vi "FaceDLControl.vi"(0 "Data In":T7 caption="Données en entrée", 2 "Display State In":T5 caption="État d'affichage en entrée", 3 "Container State":T6 caption="État du conteneur") -> (6 "Data Out":T7 caption="Données en sortie", 7 "Display State Out":T5 caption="État d'affichage en sortie", 8 "Action":T4)   [LabVIEW 2015, in "ControlDL.xctl"]
uses:
  ControlDL.xctl
  <vilib>/_xctls/Action.ctl
  <vilib>/_xctls/XControlSupport.lvlib
  <vilib>/_xctls/Container State.ctl
  DataDLControl.ctl
  stateDLControl.ctl
  controls/DLSD.ctl
  controls/DLlongVerSD.ctl
panel:
  in  "param":T1={"Short"={"min"=-100.0, "max"=48.0, "real pos"=-48.0}, "Long"={"min"=-900.0, "max"=100.0, "real pos"=-100.0}}
  in  "Enable":bool
  in  "pos long":dbl caption="pos, mm"
  in  "DL_long":T2=1.0 min=0.0 max=1.0 scale=-0.1..1.2 scale format="%.2f"
  in  "pos short":dbl caption="pos,mm"
  in  "DL_short":T3=1.0 min=0.0 max=1.0 scale format="%#_6f"
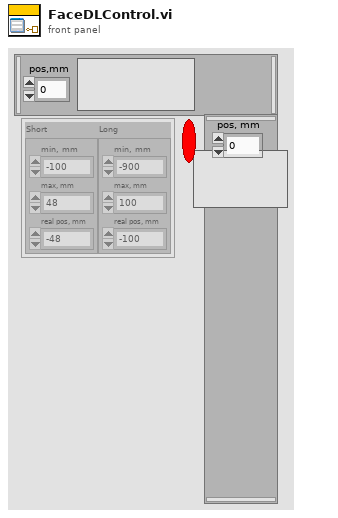
[diagram p1: front panel]
types:
  T1 = cluster{"Short":cluster{"min":dbl, "max":dbl, "real pos":dbl}, "Long":cluster{"min":dbl, "max":dbl, "real pos":dbl}}
  T2 = typedef "DLlongVerSD.ctl" = dbl
  T3 = typedef "DLSD.ctl" = dbl
  T4 = typedef "XControlSupport.lvlib/Action.ctl" = cluster{"Data Changed?":bool, "State Changed?":bool, "Action Name":string}
  T5 = typedef "ControlDL.xctl/stateDLControl.ctl" = cluster{"param":cluster{"Short":cluster{"min":dbl, "max":dbl, "real pos":dbl}, "Long":cluster{"min":dbl, "max":dbl, "real pos":dbl}}, "pos short":dbl, "pos Long":dbl, "DLmove_short":refnum<user-event>, "DLmove_long":refnum<user-event>}
  T6 = typedef "XControlSupport.lvlib/Container State.ctl" = cluster{"Indicator?":bool, "Run Mode?":bool, " Refnum":refnum<vi>}
  T7 = typedef "ControlDL.xctl/DataDLControl.ctl" = cluster{"pos short":dbl, "pos long":dbl}
  T8 = enum8{"Enabled", "Disabled", "Disabled and Grayed Out"}
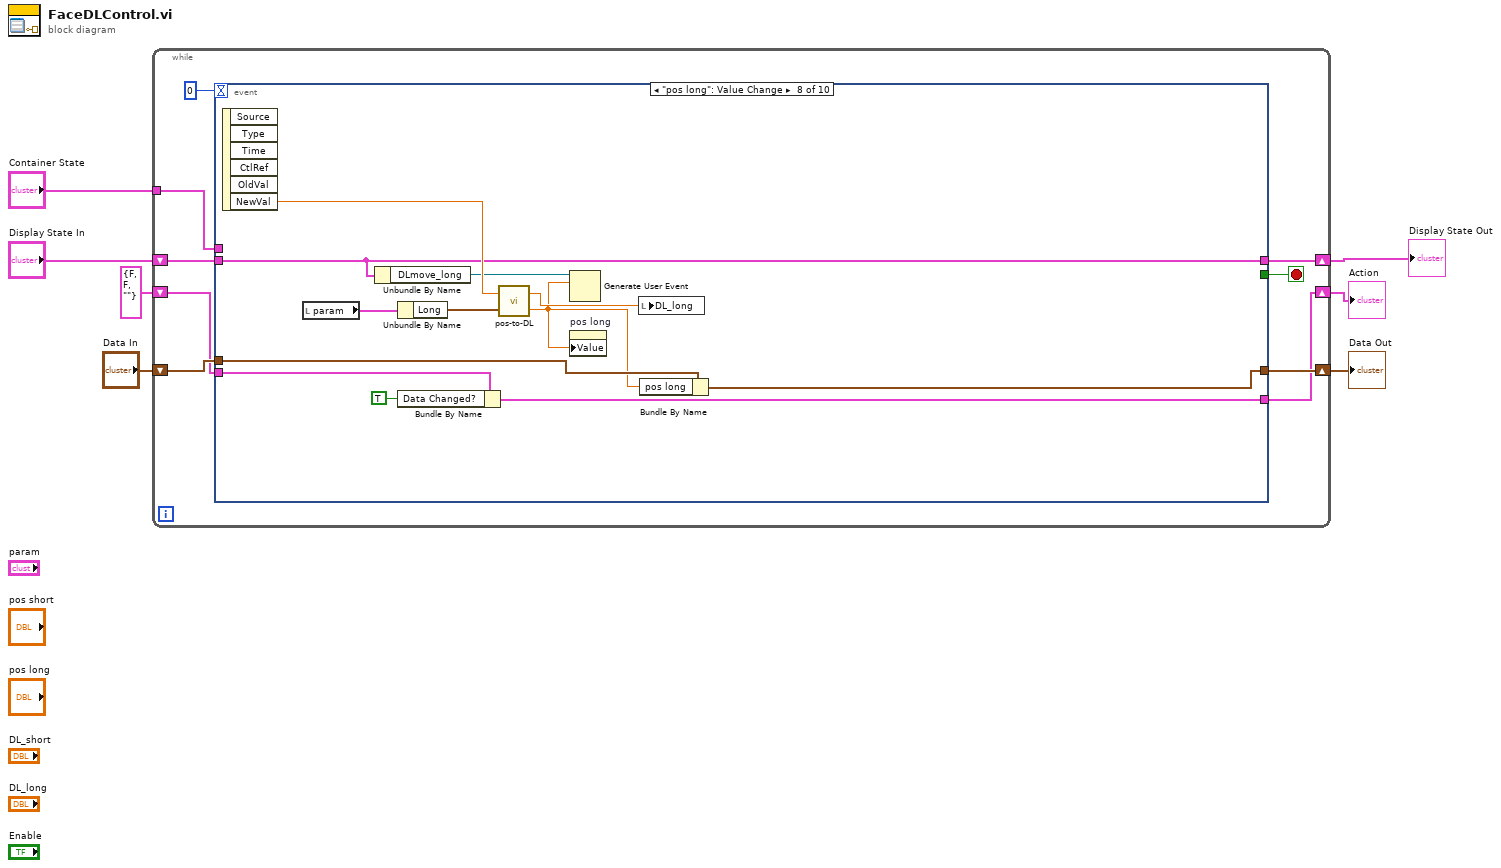
[diagram p0: block diagram]
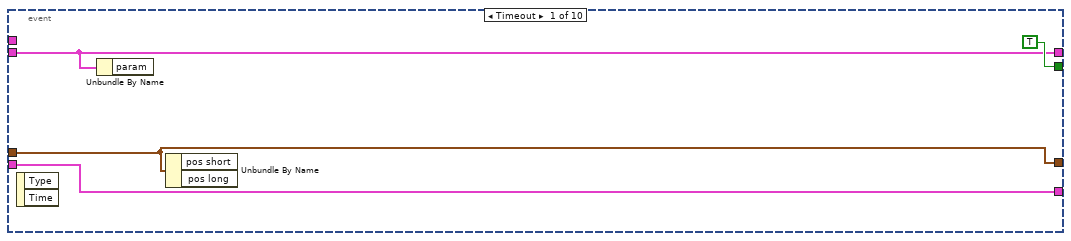
[diagram p2: hidden frame]
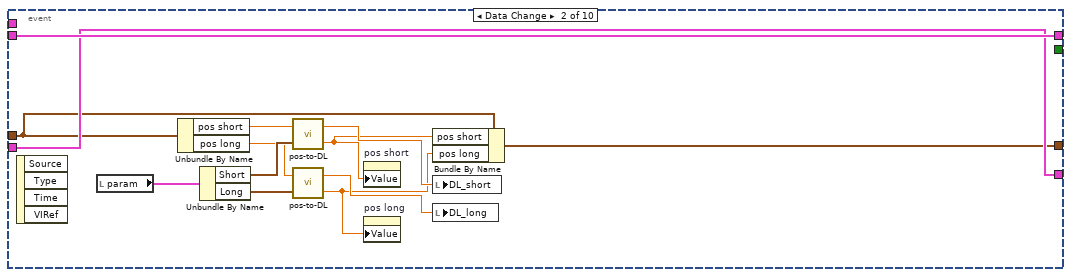
[diagram p3: hidden frame]
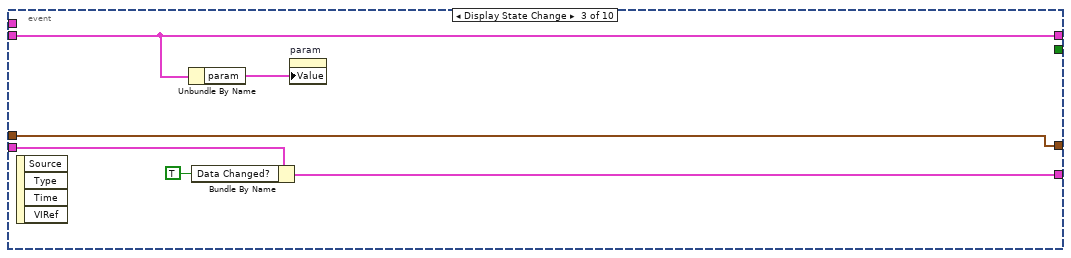
[diagram p4: hidden frame]
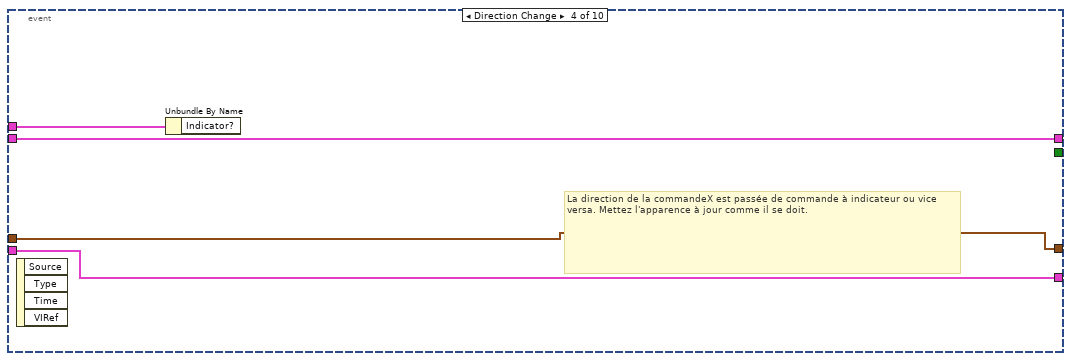
[diagram p5: hidden frame]
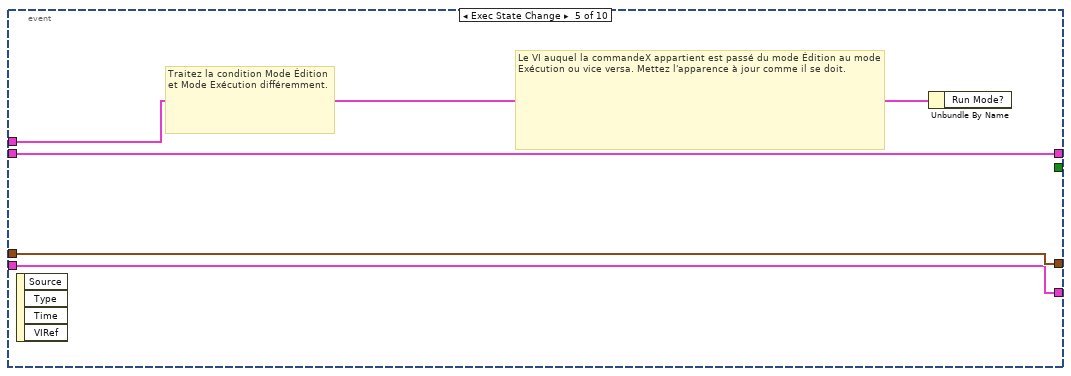
[diagram p6: hidden frame]
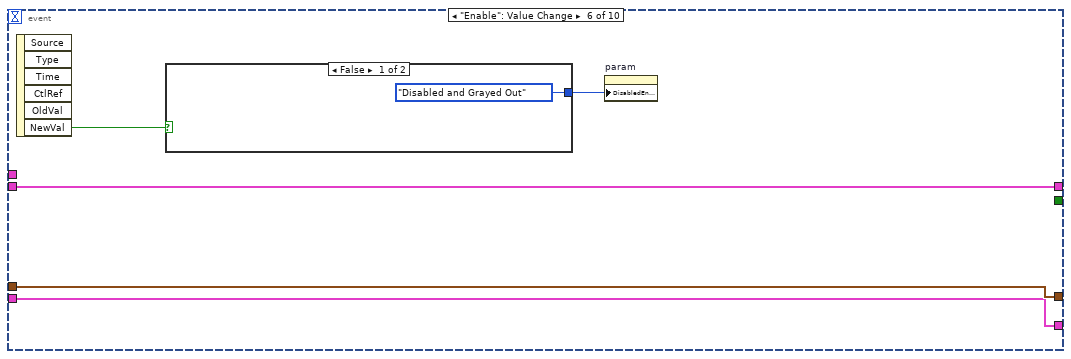
[diagram p7: hidden frame]
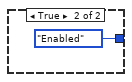
[diagram p8: hidden frame]
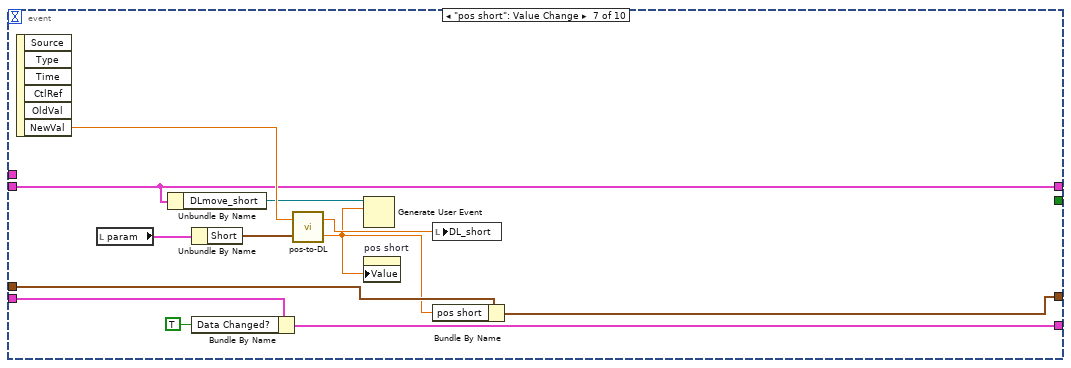
[diagram p9: hidden frame]
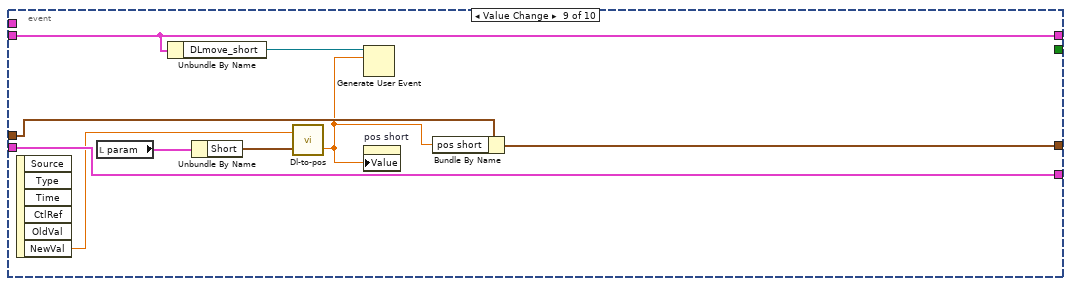
[diagram p10: hidden frame]
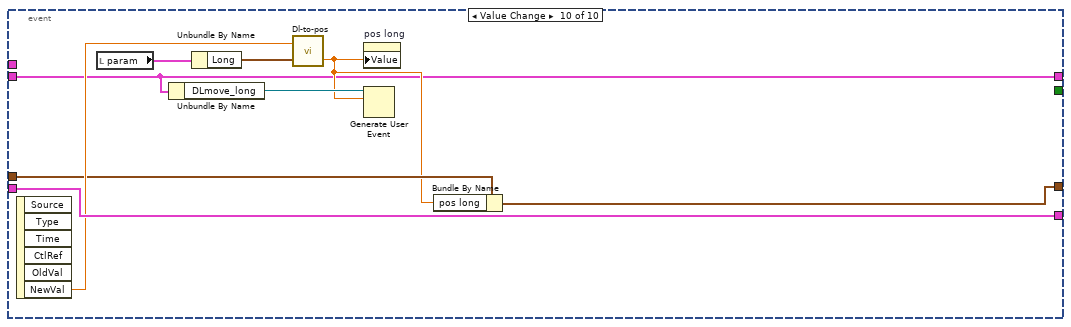
[diagram p11: hidden frame]
diagram:
  n1 = while {
    shift-right: [w15] -> w4
    shift-left: "Display State In" -> [w16]
    tunnel: "Container State" -> [w12]
    shift-right: [w10] -> w7
    shift-left: "Data In" -> [w11]
    shift-right: [w8] -> w2
    shift-left: T4 {"Data Changed?"=FALSE, "State Changed?"=FALSE, "Action Name"=""} ("Action") -> [w9]
    stop <- w14 stop-if-true
    n2 = event shown="[7] \"pos long\": Value Change" {
      selector: _ -> [_ _ _ _ _ _ _ _ _ _]
      dyn-events: _ -> [_ _ _ _ _ _ _ _ _ _]
      timeout: 0 -> [_ _ _ _ _ _ _ _ _ _]
      tunnel: w16 -> [w18 w33 w37 w42 w46 w52 w57 w67 w79 w88]
      tunnel: [w18 w33 w37 w42 w46 w52 w57 w67 w79 w88] -> w15
      tunnel: [TRUE _ _ _ _ _ _ _ _ _] -> w14
      tunnel: w12 -> [_ _ _ w43 w47 _ _ _ _ _]
      tunnel: w11 -> [w17 w26 w39 w41 w45 w51 w61 w73 w83 w92]
      tunnel: [w17 w27 w39 w41 w45 w51 w60 w72 w82 w91] -> w10
      tunnel: [w19 w32 w35 w40 w44 w50 w65 w77 w87 w96] -> w8
      tunnel: w9 -> [w19 w32 w36 w40 w44 w50 w66 w78 w87 w96]
      event Timeout {
        n3 = event-data() -> ()  [unwired: 1 in, 2 out]
        n4 = Unbundle By Name(w18) -> ()  [unwired: 1 out]
        n5 = Unbundle By Name(w17) -> ()  [unwired: 2 out]
      }
      event Data Change {
        n6 = event-data() -> ()  [unwired: 1 in, 4 out]
        n7 = local read "param"() -> (w31:T1)
        n8 = Unbundle By Name(w26) -> ("pos short"=w23:dbl, "pos long"=w24:dbl)
        n9 = Unbundle By Name(w31) -> ("Short"=w30:cluster{"min":dbl, "max":dbl, "real pos":dbl}, "Long"=w25:cluster{"min":dbl, "max":dbl, "real pos":dbl})
        n10 = call "pos-to-DL.vi"("DL param"=w30, "pos, mm"=w23) -> ("pos, mm"=w21:dbl, "DL pos"=w29:dbl)
        n11 = call "pos-to-DL.vi"("DL param"=w25, "pos, mm"=w24) -> ("pos, mm"=w22:dbl, "DL pos"=w28:dbl)
        n12 = property on="pos short" class="DigNum (strict)"("Value"=w21) -> ()  [unwired: 2 in, 2 out]
        n13 = property on="pos long" class="DigNum (strict)"("Value"=w22) -> ()  [unwired: 2 in, 2 out]
        n14 = Bundle By Name(cluster=w26, "pos short"=w21, "pos long"=w22) -> (w27:T7)
        n15 = local write "DL_short"(w29) -> ()
        n16 = local write "DL_long"(w28) -> ()
      }
      event Display State Change {
        n17 = event-data() -> ()  [unwired: 1 in, 4 out]
        n18 = Unbundle By Name(w37) -> ("param"=w38:T1)
        n19 = Bundle By Name(cluster=w36, "Data Changed?"=TRUE) -> (w35:T4)
        n20 = property on="param" class="Clust (strict)"("Value"=w38) -> ()  [unwired: 2 in, 2 out]
      }
      event Direction Change {
        # "La direction de la commandeX est passée de commande à indicateur ou vice versa. Mettez l'apparence à jour comme il se doit."
        n21 = event-data() -> ()  [unwired: 1 in, 4 out]
        n22 = Unbundle By Name(w43) -> ()  [unwired: 1 out]
      }
      event Exec State Change {
        # "Le VI auquel la commandeX appartient est passé du mode Édition au mode Exécution ou vice versa. Mettez l'apparence à jour comme il se doit."
        # "Traitez la condition Mode Édition et Mode Exécution différemment."
        n23 = event-data() -> ()  [unwired: 1 in, 4 out]
        n24 = Unbundle By Name(w47) -> ()  [unwired: 1 out]
      }
      event "Enable": Value Change {
        n25 = event-data() -> ("NewVal"=w49:bool)  [unwired: 1 in, 5 out]
        n26 = case shown="False" w49 {
          tunnel: [T8."Disabled and Grayed Out" ("Disabled") T8."Enabled" ("Disabled")] -> w48
          frame False {
          }
          frame True {
          }
        }
        n27 = property on="param" class="Clust (strict)"("DisabledEnum"=w48) -> ()  [unwired: 2 in, 2 out]
      }
      event "pos short": Value Change {
        n28 = event-data() -> ("NewVal"=w59:dbl)  [unwired: 1 in, 5 out]
        n29 = local read "param"() -> (w63:T1)
        n30 = Unbundle By Name(w57) -> ("DLmove_short"=w56:refnum<user-event>)
        n31 = Unbundle By Name(w63) -> ("Short"=w62:cluster{"min":dbl, "max":dbl, "real pos":dbl})
        n32 = Bundle By Name(cluster=w66, "Data Changed?"=TRUE ("State Changed?")) -> (w65:T4)
        n33 = call "pos-to-DL.vi"("DL param"=w62, "pos, mm"=w59) -> ("pos, mm"=w55:dbl, "DL pos"=w58:dbl)
        n34 = Generate User Event(user event=w56, event data cluster=w55) -> ()  [unwired: 2 in, 2 out]
        n35 = property on="pos short" class="DigNum (strict)"("Value"=w55) -> ()  [unwired: 2 in, 2 out]
        n36 = local write "DL_short"(w58) -> ()
        n37 = Bundle By Name(cluster=w61, "pos short"=w55) -> (w60:T7)
      }
      event "pos long": Value Change {
        n38 = event-data() -> ("NewVal"=w71:dbl)  [unwired: 1 in, 5 out]
        n39 = local read "param"() -> (w75:T1)
        n40 = Unbundle By Name(w67) -> ("DLmove_long"=w69:refnum<user-event>)
        n41 = Unbundle By Name(w75) -> ("Long"=w74:cluster{"min":dbl, "max":dbl, "real pos":dbl})
        n42 = Bundle By Name(cluster=w78, "Data Changed?"=TRUE ("State Changed?")) -> (w77:T4)
        n43 = call "pos-to-DL.vi"("DL param"=w74, "pos, mm"=w71) -> ("pos, mm"=w68:dbl, "DL pos"=w70:dbl)
        n44 = Generate User Event(user event=w69, event data cluster=w68) -> ()  [unwired: 2 in, 2 out]
        n45 = property on="pos long" class="DigNum (strict)"("Value"=w68) -> ()  [unwired: 2 in, 2 out]
        n46 = local write "DL_long"(w70) -> ()
        n47 = Bundle By Name(cluster=w73, "pos long"=w68) -> (w72:T7)
      }
      event Value Change {
        n48 = event-data() -> ("NewVal"=w84:T3)  [unwired: 1 in, 5 out]
        n49 = local read "param"() -> (w85:T1)
        n50 = Unbundle By Name(w79) -> ("DLmove_short"=w80:refnum<user-event>)
        n51 = Unbundle By Name(w85) -> ("Short"=w86:cluster{"min":dbl, "max":dbl, "real pos":dbl})
        n52 = call "Dl-to-pos.vi"("DL param"=w86, "DL_pos"=w84) -> ("pos, mm"=w81:dbl)  [unwired: 1 out]
        n53 = Generate User Event(user event=w80, event data cluster=w81) -> ()  [unwired: 2 in, 2 out]
        n54 = property on="pos short" class="DigNum (strict)"("Value"=w81) -> ()  [unwired: 2 in, 2 out]
        n55 = Bundle By Name(cluster=w83, "pos short"=w81) -> (w82:T7)
      }
      event Value Change {
        n56 = event-data() -> ("NewVal"=w93:T2)  [unwired: 1 in, 5 out]
        n57 = local read "param"() -> (w94:T1)
        n58 = Unbundle By Name(w88) -> ("DLmove_long"=w90:refnum<user-event>)
        n59 = Unbundle By Name(w94) -> ("Long"=w95:cluster{"min":dbl, "max":dbl, "real pos":dbl})
        n60 = call "Dl-to-pos.vi"("DL param"=w95, "DL_pos"=w93) -> ("pos, mm"=w89:dbl)  [unwired: 1 out]
        n61 = property on="pos long" class="DigNum (strict)"("Value"=w89) -> ()  [unwired: 2 in, 2 out]
        n62 = Generate User Event(user event=w90, event data cluster=w89) -> ()  [unwired: 2 in, 2 out]
        n63 = Bundle By Name(cluster=w92, "pos long"=w89) -> (w91:T7)
      }
    }
  }
  "Display State Out" <- w4
  "Data Out" <- w7
  "Action" <- w2
